vi "CRYAPI SPLITE.vi"(4 "tSpliter_In":T2, 6 "tFrame":T4, 8 "tSpliter":T2, 9 "sData":string, 10 "nData":i32, 11 "sAction":string) -> (0 "nData_Out":i32, 1 "tLR_Out":T1, 3 "tSpliter_Out":T2)   [LabVIEW 2013]
uses:
  <vilib>/Utility/miscctls.llb/LVRectTypeDef.ctl
  CRYMain Sub Window Global.vi
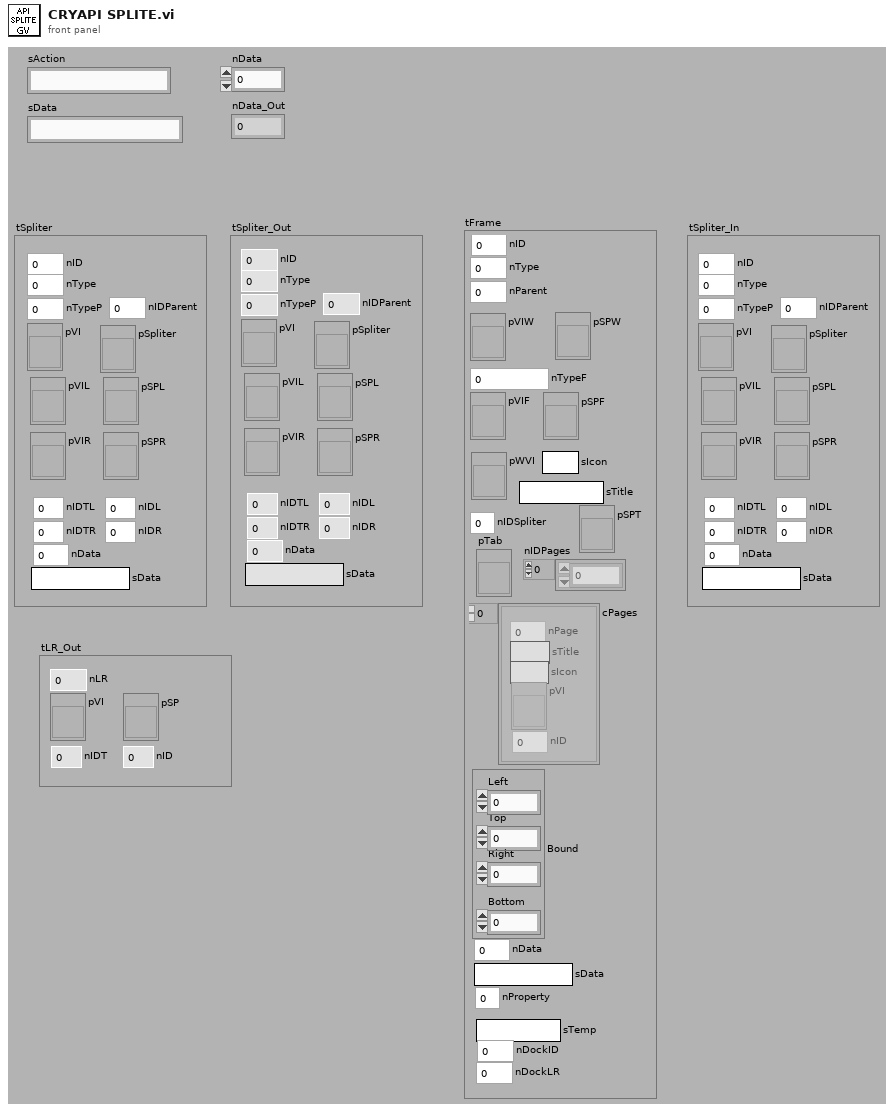
[diagram p1: front panel]
types:
  T1 = cluster{"pSP":refnum<vi>, "pVI":refnum<vi>, "nIDT":i32, "nID":i32, "nLR":i32}
  T2 = cluster{"nType":i32, "nTypeP":i32, "pVI":refnum<vi>, "pSpliter":refnum<vi>, "pSPL":refnum<vi>, "pVIL":refnum<vi>, "pSPR":refnum<vi>, "pVIR":refnum<vi>, "nIDTL":i32, "nIDL":i32, "nIDTR":i32, "nIDR":i32, "nID":i32, "nIDParent":i32, "nData":i32, "sData":string}
  T3 = typedef "LVRectTypeDef.ctl" = cluster{"Left":i16, "Top":i16, "Right":i16, "Bottom":i16}
  T4 = cluster{"nType":i32, "nParent":i32, "pVIW":refnum<vi>, "pSPW":refnum<vi>, "nTypeF":i32, "pVIF":refnum<vi>, "pSPF":refnum<vi>, "nIDSpliter":i32, "nProperty":i32, "Bound":T3, "nID":i32, "nData":i32, "sData":string, "pWVI":refnum<vi>, "sTitle":string, "cPages":cluster{"nPage":i32, "sTitle":string, "sIcon":string, "pVI":refnum<vi>, "nID":i32}[], "pTab":refnum<vi>, "nIDPages":i32[], "pSPT":refnum<vi>, "sTemp":string, "nDockID":i32, "nDockLR":i32, "sIcon":string}
  T5 = enum16{"Sticks Top/Left", "Sticks Bottom/Right", "Proportional"}
  T6 = cluster{"nID":i32, "sTiltle":string, "pVI":refnum<vi>, "pSP":refnum<vi>, "pTab":refnum<vi>, "pSPT":refnum<vi>, "nWinType":i32, "sIcon":string}
  T7 = cluster{"nID":i32[], "Spliter":cluster{"nType":i32, "nTypeP":i32, "pVI":refnum<vi>, "pSpliter":refnum<vi>, "pSPL":refnum<vi>, "pVIL":refnum<vi>, "pSPR":refnum<vi>, "pVIR":refnum<vi>, "nIDTL":i32, "nIDL":i32, "nIDTR":i32, "nIDR":i32, "nID":i32, "nIDParent":i32, "nData":i32, "sData":string}[]}
  T8 = cluster{"nType":i32, "nTypeP":i32, "pVI":refnum<vi>, "pSpliter":refnum<vi>, "pSPL":refnum<vi>, "pVIL":refnum<vi>, "pSPR":refnum<vi>, "pVIR":refnum<vi>, "nIDTL":i32, "nIDL":i32, "nIDTR":i32, "nIDR":i32, "nID":i32, "nIDParent":i32, "nData":i32, "sData":string}[]
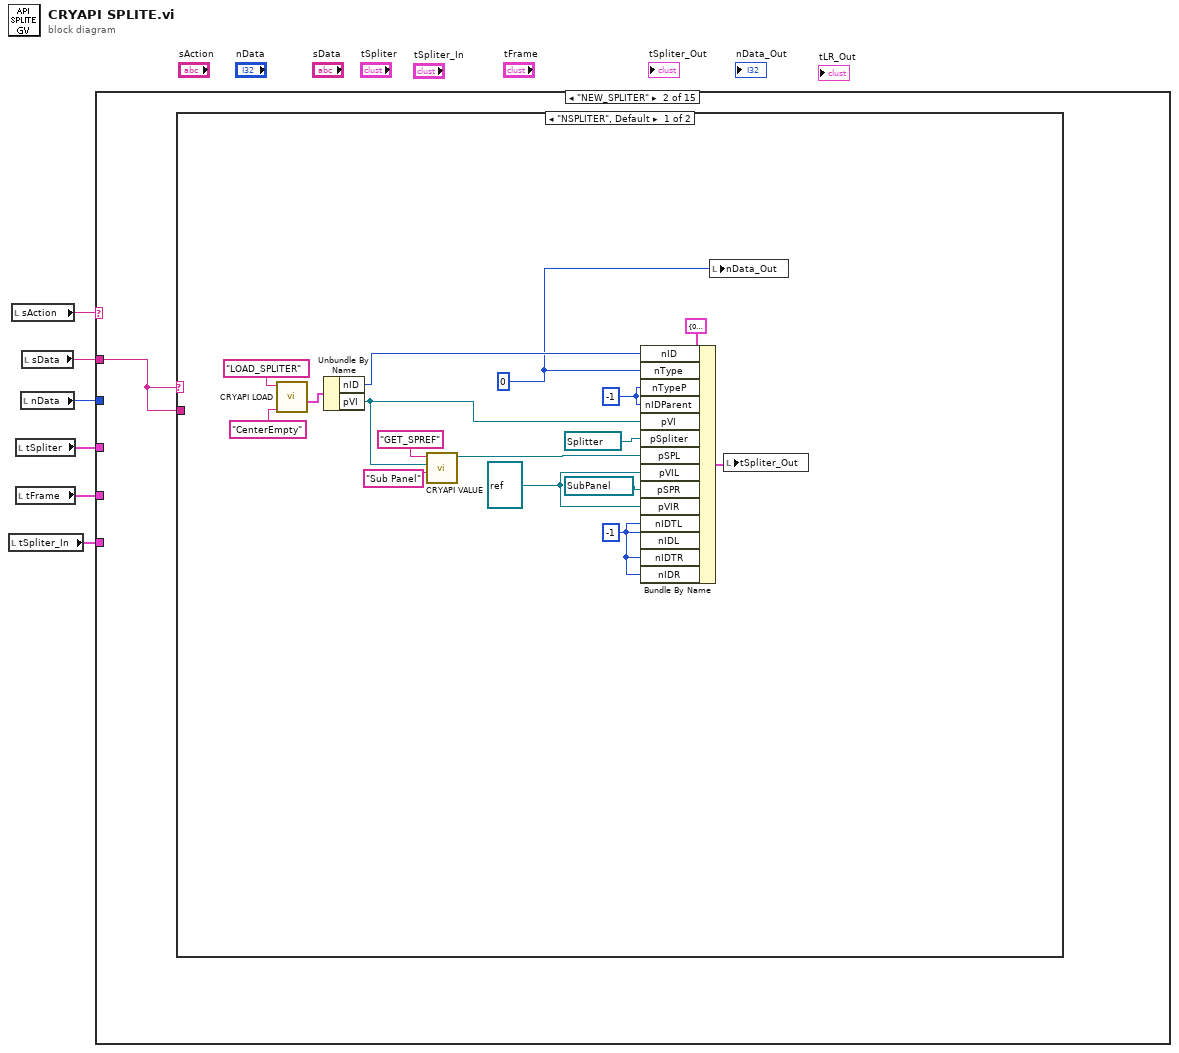
[diagram p0: block diagram]
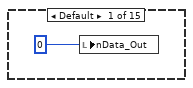
[diagram p2: hidden frame]
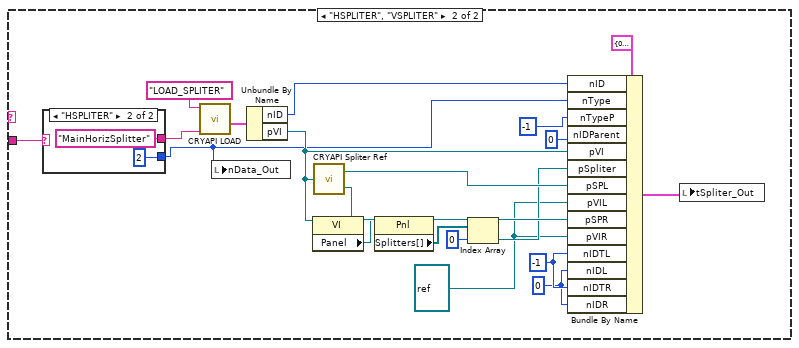
[diagram p3: hidden frame]
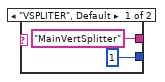
[diagram p4: hidden frame]
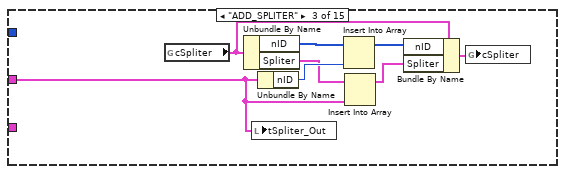
[diagram p5: hidden frame]
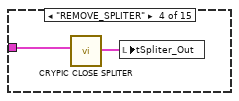
[diagram p6: hidden frame]
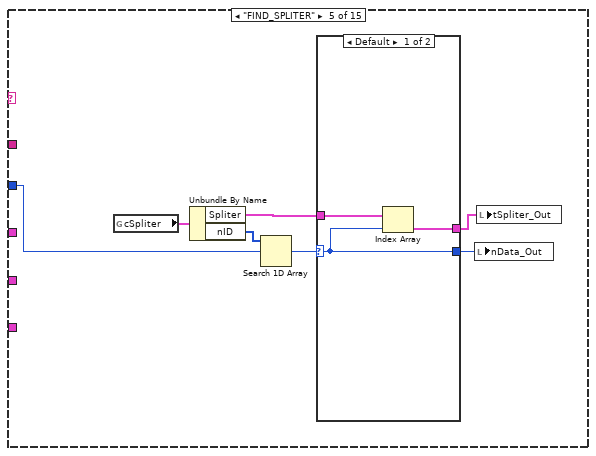
[diagram p7: hidden frame]
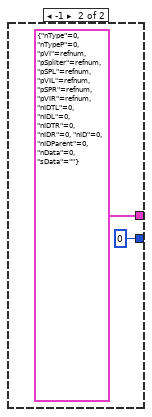
[diagram p8: hidden frame]
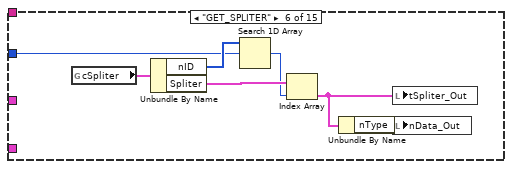
[diagram p9: hidden frame]
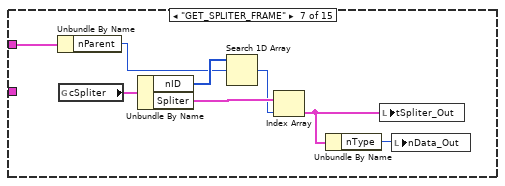
[diagram p10: hidden frame]
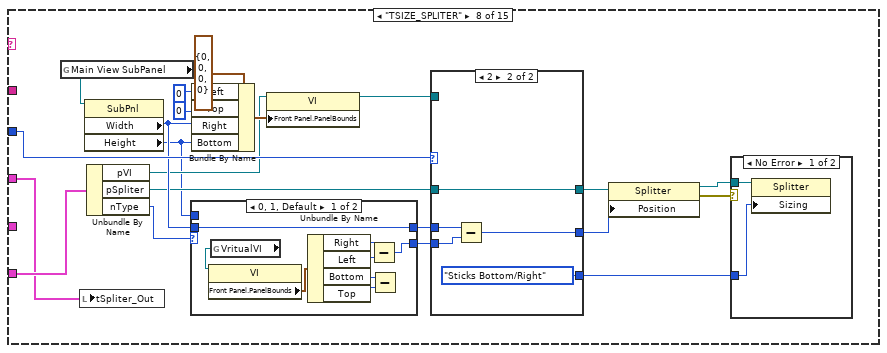
[diagram p11: hidden frame]
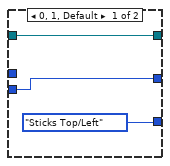
[diagram p13: hidden frame]
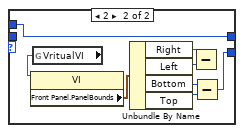
[diagram p14: hidden frame]
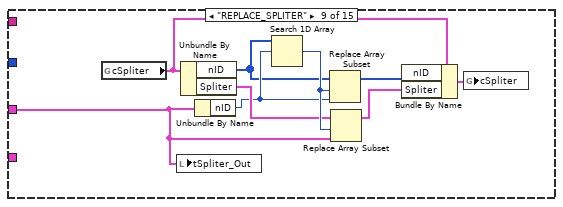
[diagram p15: hidden frame]
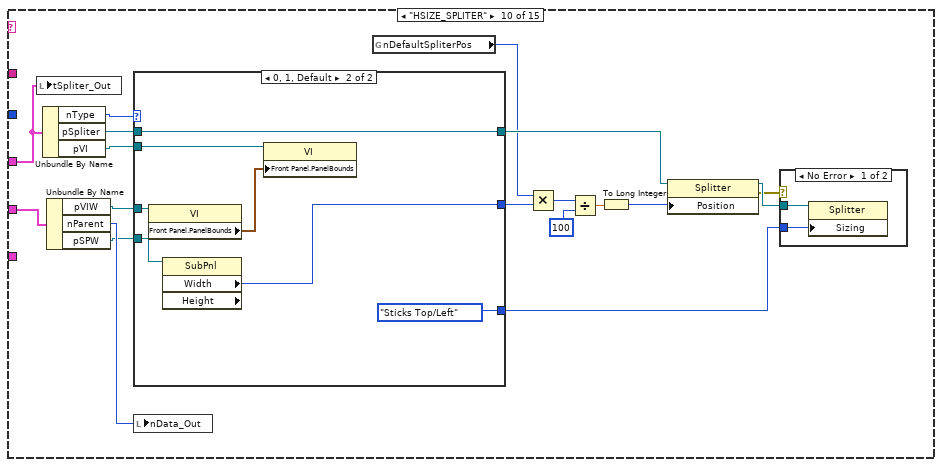
[diagram p16: hidden frame]
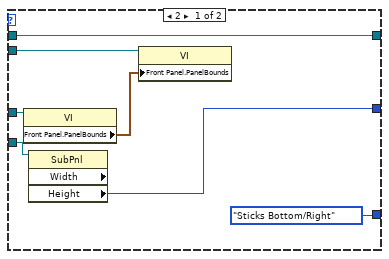
[diagram p18: hidden frame]
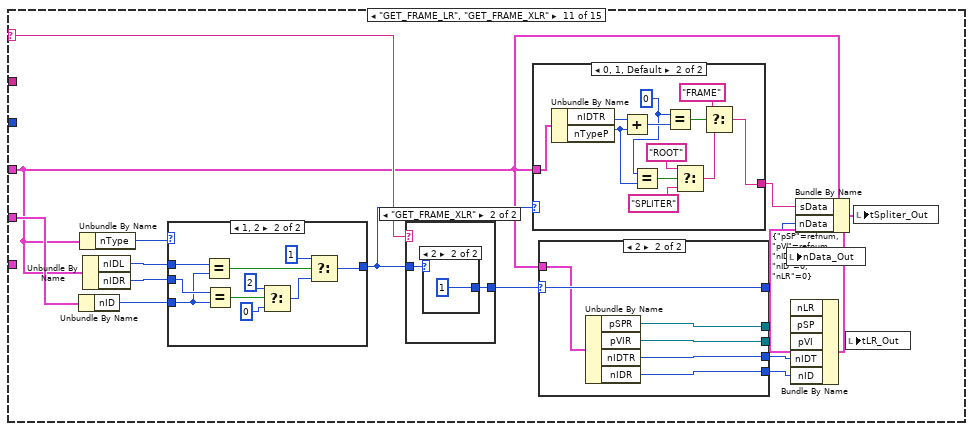
[diagram p19: hidden frame]
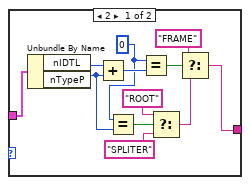
[diagram p20: hidden frame]
diagram:
  n1 = local read "tSpliter_In"() -> (w1:T2)
  n2 = local read "sAction"() -> (w6:string)
  n3 = local read "tSpliter"() -> (w4:T2)
  n4 = local read "tFrame"() -> (w2:T4)
  n5 = local read "nData"() -> (w3:i32)
  n6 = local read "sData"() -> (w5:string)
  n7 = case shown="\"NEW_SPLITER\"" w6 {
    selector: w6 -> [_ _ _ _ _ _ _ _ _ _ w181 w252 w322 w391 _]
    tunnel: w5 -> [_ w8 _ _ _ _ _ _ _ _ _ _ _ w389 w443]
    tunnel: w4 -> [_ _ w49 w58 _ _ _ w86 w133 w156 w176 w248 w319 w390 _]
    tunnel: w3 -> [_ _ _ _ w64 w74 _ w100 _ _ _ _ w316 w388 w448]
    tunnel: w2 -> [_ _ _ _ _ _ w79 _ _ w151 w189 _ _ _ w444]
    tunnel: w1 -> [_ _ _ _ _ _ _ w87 _ _ _ w249 _ _ _]
    frame Default {
      n8 = local write "nData_Out"(0 ("nData_Out")) -> ()
    }
    frame "NEW_SPLITER" {
      n9 = case shown="\"NSPLITER\", Default" w8 {
        tunnel: w8 -> [_ w41]
        frame "NSPLITER", Default {
          w19 = -1
          w20 = refnum<vi> refnum ("pVIL")
          w16 = -1 ("nParent")
          w10 = 0
          n10 = call "CRYAPI LOAD.vi"("sData"="CenterEmpty" ("sAction"), "sAction"="LOAD_SPLITER") -> ("tWindow_Out"=w22:T6)  [unwired: 4 in, 5 out]
          n11 = Unbundle By Name(w22) -> ("nID"=w21:i32, "pVI"=w12:refnum<vi>)
          n12 = call "CRYAPI VALUE.vi"("sControlName"="Sub Panel", "pVIRef"=w12, "sAction"="GET_SPREF") -> ("pSPRef"=w11:refnum<vi>)  [unwired: 2 in, 6 out]
          n13 = Bundle By Name(cluster=T2 {"nType"=0, "nTypeP"=0, "pVI"=refnum, "pSpliter"=refnum, "pSPL"=refnum, "pVIL"=refnum, "pSPR"=refnum, "pVIR"=refnum, "nIDTL"=0, "nIDL"=0, "nIDTR"=0, "nIDR"=0, "nID"=0, "nIDParent"=0, "nData"=0, "sData"=""} ("tSpliter_Out"), "nID"=w21, "nType"=w10, "nTypeP"=w16, "nIDParent"=w16, "pVI"=w12, "pSpliter"=refnum<vi> refnum, "pSPL"=w11, "pVIL"=w20, "pSPR"=refnum<vi> refnum, "pVIR"=w20, "nIDTL"=w19, "nIDL"=w19, "nIDTR"=w19, "nIDR"=w19) -> (w24:T2)
          n14 = local write "nData_Out"(w10) -> ()
          n15 = local write "tSpliter_Out"(w24) -> ()
        }
        frame "HSPLITER", "VSPLITER" {
          w28 = 0
          w32 = -1
          w33 = refnum<vi> refnum ("pVIL")
          n16 = case shown="\"HSPLITER\"" w41 {
            tunnel: ["MainVertSplitter" ("sAction") "MainHorizSplitter" ("sAction")] -> w42
            tunnel: [1 2] -> w29
            frame "VSPLITER", Default {
            }
            frame "HSPLITER" {
            }
          }
          n17 = call "CRYAPI LOAD.vi"("sData"=w42, "sAction"="LOAD_SPLITER") -> ("tWindow_Out"=w43:T6)  [unwired: 4 in, 5 out]
          n18 = local write "nData_Out"(w29) -> ()
          n19 = Unbundle By Name(w43) -> ("nID"=w34:i32, "pVI"=w31:refnum<vi>)
          n20 = property class="VI"(reference=w31) -> ("Panel"=w36:refnum<vi>)  [unwired: 1 in, 2 out]
          n21 = call "CRYAPI Spliter Ref.vi"("VI Refnum"=w31) -> ("Left/Upper"=w40:refnum<vi>, "Right/Lower"=w39:refnum<vi>)
          n22 = property class="Pnl"(reference=w36) -> ("Splitters[]"=w37:refnum<vi>[])  [unwired: 1 in, 2 out]
          n23 = Index Array(array=w37, index=0) -> (element=w35:refnum<vi>)
          n24 = Bundle By Name(cluster=T2 {"nType"=0, "nTypeP"=0, "pVI"=refnum, "pSpliter"=refnum, "pSPL"=refnum, "pVIL"=refnum, "pSPR"=refnum, "pVIR"=refnum, "nIDTL"=0, "nIDL"=0, "nIDTR"=0, "nIDR"=0, "nID"=0, "nIDParent"=0, "nData"=0, "sData"=""} ("tSpliter_Out"), "nID"=w34, "nType"=w29, "nTypeP"=-1 ("nParent"), "nIDParent"=0 ("nParent"), "pVI"=w31, "pSpliter"=w35, "pSPL"=w40, "pVIL"=w33, "pSPR"=w39, "pVIR"=w33, "nIDTL"=w32, "nIDL"=w28, "nIDTR"=w32, "nIDR"=w28) -> (w25:T2)
          n25 = local write "tSpliter_Out"(w25) -> ()
        }
      }
    }
    frame "ADD_SPLITER" {
      n26 = global read "CRYMain Sub Window Global.vi" "cSpliter"() -> (w53:T7)
      n27 = Unbundle By Name(w53) -> ("nID"=w50:i32[], "Spliter"=w51:T8)
      n28 = local write "tSpliter_Out"(w49) -> ()
      n29 = Unbundle By Name(w49) -> ("nID"=w52:i32)
      n30 = Insert Into Array(array=w50, new element=w52) -> (w54:i32[])  [unwired: 1 in]
      n31 = Insert Into Array(array=w51, new element=w49) -> (w55:T8)  [unwired: 1 in]
      n32 = Bundle By Name(cluster=w53, "nID"=w54, "Spliter"=w55) -> (w56:T7)
      n33 = global write "CRYMain Sub Window Global.vi" "cSpliter"(w56) -> ()
    }
    frame "REMOVE_SPLITER" {
      n34 = call "CRYPIC CLOSE SPLITER.vi"("tSpliter"=w58) -> ("tSpliter_Out"=w57:T2)  [unwired: 10 in]
      n35 = local write "tSpliter_Out"(w57) -> ()
    }
    frame "FIND_SPLITER" {
      n36 = global read "CRYMain Sub Window Global.vi" "cSpliter"() -> (w62:T7)
      n37 = Unbundle By Name(w62) -> ("Spliter"=w61:T8, "nID"=w65:i32[])
      n38 = Search 1D Array(1D array=w65, element=w64) -> (index of element=w63:i32)  [unwired: 1 out]
      n39 = case shown="Default" w63 {
        selector: w63 -> [w66 _]
        tunnel: w61 -> [w68 _]
        tunnel: [w67 T2 {"nType"=0, "nTypeP"=0, "pVI"=refnum, "pSpliter"=refnum, "pSPL"=refnum, "pVIL"=refnum, "pSPR"=refnum, "pVIR"=refnum, "nIDTL"=0, "nIDL"=0, "nIDTR"=0, "nIDR"=0, "nID"=0, "nIDParent"=0, "nData"=0, "sData"=""} ("tSpliter")] -> w59
        tunnel: [w66 0 ("index of element")] -> w60
        frame Default {
          n40 = Index Array(array=w68, index=w66) -> (element=w67:T2)
        }
        frame -1 {
        }
      }
      n41 = local write "nData_Out"(w60) -> ()
      n42 = local write "tSpliter_Out"(w59) -> ()
    }
    frame "GET_SPLITER" {
      n43 = global read "CRYMain Sub Window Global.vi" "cSpliter"() -> (w77:T7)
      n44 = Unbundle By Name(w77) -> ("nID"=w75:i32[], "Spliter"=w76:T8)
      n45 = Search 1D Array(1D array=w75, element=w74) -> (index of element=w73:i32)  [unwired: 1 out]
      n46 = Index Array(array=w76, index=w73) -> (element=w72:T2)
      n47 = Unbundle By Name(w72) -> ("nType"=w71:i32)
      n48 = local write "tSpliter_Out"(w72) -> ()
      n49 = local write "nData_Out"(w71) -> ()
    }
    frame "GET_SPLITER_FRAME" {
      n50 = Unbundle By Name(w79) -> ("nParent"=w78:i32)
      n51 = global read "CRYMain Sub Window Global.vi" "cSpliter"() -> (w85:T7)
      n52 = Unbundle By Name(w85) -> ("nID"=w83:i32[], "Spliter"=w84:T8)
      n53 = Search 1D Array(1D array=w83, element=w78) -> (index of element=w82:i32)  [unwired: 1 out]
      n54 = Index Array(array=w84, index=w82) -> (element=w81:T2)
      n55 = Unbundle By Name(w81) -> ("nType"=w80:i32)
      n56 = local write "tSpliter_Out"(w81) -> ()
      n57 = local write "nData_Out"(w80) -> ()
    }
    frame "TSIZE_SPLITER" {
      n58 = global read "CRYMain Sub Window Global.vi" "Main View SubPanel"() -> (w106:refnum<vi>)
      n59 = local write "tSpliter_Out"(w86) -> ()
      n60 = property class="SubPnl"(reference=w106) -> ("Width"=w98:u32, "Height"=w93:u32)  [unwired: 1 in, 2 out]
      n61 = Unbundle By Name(w87) -> ("pVI"=w95:refnum<vi>, "pSpliter"=w94:refnum<vi>, "nType"=w101:i32)
      n62 = case shown="0, 1, Default" w101 {
        tunnel: [w118 w126] -> w99
        tunnel: w93 -> [_ w125]
        tunnel: w98 -> [w117 _]
        tunnel: [w117 w125] -> w97
        frame 0, 1, Default {
          n63 = global read "CRYMain Sub Window Global.vi" "VritualVI"() -> (w124:refnum<vi>)
          n64 = property class="VI"(reference=w124) -> ("Front Panel.PanelBounds"=w123:T3)  [unwired: 1 in, 2 out]
          n65 = Unbundle By Name(w123) -> ("Right"=w122:i16, "Left"=w121:i16, "Bottom"=w120:i16, "Top"=w119:i16)
          n66 = Subtract(x=w122, y=w121) -> (x-y=w118:i16)
          n67 = Subtract(x=w120, y=w119) -> ()  [unwired: 1 out]
        }
        frame 2 {
          n68 = global read "CRYMain Sub Window Global.vi" "VritualVI"() -> (w132:refnum<vi>)
          n69 = property class="VI"(reference=w132) -> ("Front Panel.PanelBounds"=w131:T3)  [unwired: 1 in, 2 out]
          n70 = Unbundle By Name(w131) -> ("Right"=w130:i16, "Left"=w129:i16, "Bottom"=w128:i16, "Top"=w127:i16)
          n71 = Subtract(x=w130, y=w129) -> ()  [unwired: 1 out]
          n72 = Subtract(x=w128, y=w127) -> (x-y=w126:i16)
        }
      }
      n73 = Bundle By Name(cluster=T3 {"Left"=0, "Top"=0, "Right"=0, "Bottom"=0} ("Bound_Out"), "Left"=i16 0, "Top"=i16 0, "Right"=w98, "Bottom"=w93) -> (w105:T3)
      n74 = property class="VI"(reference=w95, "Front Panel.PanelBounds"=w105) -> (reference out=w96:refnum<vi>)  [unwired: 1 in, 1 out]
      n75 = case shown="2" w100 {
        tunnel: w99 -> [w111 w115]
        tunnel: [w111 w114] -> w91
        tunnel: w97 -> [_ w116]
        tunnel: w96 -> [_ _]
        tunnel: w94 -> [w110 w113]
        tunnel: [w110 w113] -> w92
        tunnel: [T5."Sticks Top/Left" ("Sizing") T5."Sticks Bottom/Right" ("Sizing")] -> w88
        frame 0, 1, Default {
        }
        frame 2 {
          n76 = Subtract(x=w116, y=w115) -> (x-y=w114:u32)
        }
      }
      n77 = property class="Splitter"(reference=w92, "Position"=w91) -> (reference out=w89:refnum<vi>, error out=w90:errorcluster)  [unwired: 1 in]
      n78 = case shown="No Error" w90 {
        tunnel: w88 -> [w108 _]
        tunnel: w89 -> [w107 _]
        frame No Error {
          n79 = property class="Splitter"(reference=w107, "Sizing"=w108) -> ()  [unwired: 1 in, 2 out]
        }
        frame Error {
        }
      }
    }
    frame "REPLACE_SPLITER" {
      n80 = global read "CRYMain Sub Window Global.vi" "cSpliter"() -> (w136:T7)
      n81 = local write "tSpliter_Out"(w133) -> ()
      n82 = Unbundle By Name(w136) -> ("nID"=w137:i32[], "Spliter"=w140:T8)
      n83 = Unbundle By Name(w133) -> ("nID"=w138:i32)
      n84 = Search 1D Array(1D array=w137, element=w138) -> (index of element=w141:i32)  [unwired: 1 out]
      n85 = Replace Array Subset(array=w137, new element=w138, index=w141) -> (w135:i32[])
      n86 = Replace Array Subset(array=w140, new element=w133, index=w141) -> (w139:T8)
      n87 = Bundle By Name(cluster=w136, "nID"=w135, "Spliter"=w139) -> (w134:T7)
      n88 = global write "CRYMain Sub Window Global.vi" "cSpliter"(w134) -> ()
    }
    frame "HSIZE_SPLITER" {
      n89 = local write "tSpliter_Out"(w156) -> ()
      n90 = Unbundle By Name(w156) -> ("nType"=w152:i32, "pSpliter"=w154:refnum<vi>, "pVI"=w155:refnum<vi>)
      n91 = Unbundle By Name(w151) -> ("pVIW"=w159:refnum<vi>, "nParent"=w150:i32, "pSPW"=w149:refnum<vi>)
      n92 = case shown="0, 1, Default" w152 {
        tunnel: w159 -> [w168 w175]
        tunnel: [w163 w170] -> w146
        tunnel: w155 -> [w167 w174]
        tunnel: w154 -> [w165 w172]
        tunnel: [w165 w172] -> w153
        tunnel: w149 -> [w164 w171]
        tunnel: [T5."Sticks Bottom/Right" ("Sizing") T5."Sticks Top/Left" ("Sizing")] -> w148
        frame 2 {
          n93 = property class="VI"(reference=w168) -> ("Front Panel.PanelBounds"=w166:T3)  [unwired: 1 in, 2 out]
          n94 = property class="SubPnl" props=["Width", "Height"](reference=w164) -> ("Height"=w163:u32)  [unwired: 1 in, 3 out]
          n95 = property class="VI"(reference=w167, "Front Panel.PanelBounds"=w166) -> ()  [unwired: 1 in, 2 out]
        }
        frame 0, 1, Default {
          n96 = property class="VI"(reference=w175) -> ("Front Panel.PanelBounds"=w173:T3)  [unwired: 1 in, 2 out]
          n97 = property class="SubPnl" props=["Width", "Height"](reference=w171) -> ("Width"=w170:u32)  [unwired: 1 in, 3 out]
          n98 = property class="VI"(reference=w174, "Front Panel.PanelBounds"=w173) -> ()  [unwired: 1 in, 2 out]
        }
      }
      n99 = local write "nData_Out"(w150) -> ()
      n100 = global read "CRYMain Sub Window Global.vi" "nDefaultSpliterPos"() -> (w147:i32)
      n101 = Multiply(x=w147, y=w146) -> (x*y=w145:u32)
      n102 = Divide(x=w145, y=u32 100) -> (x/y=w143:dbl)
      n103 = To Long Integer(number=w143) -> (32bit integer=w142:i32)
      n104 = property class="Splitter"(reference=w153, "Position"=w142) -> (reference out=w158:refnum<vi>, error out=w157:errorcluster)  [unwired: 1 in]
      n105 = case shown="No Error" w157 {
        tunnel: w158 -> [w161 _]
        tunnel: w148 -> [w160 _]
        frame No Error {
          n106 = property class="Splitter"(reference=w161, "Sizing"=w160) -> ()  [unwired: 1 in, 2 out]
        }
        frame Error {
        }
      }
    }
    frame "GET_FRAME_LR", "GET_FRAME_XLR" {
      n107 = Unbundle By Name(w189) -> ("nID"=w191:i32)
      n108 = Unbundle By Name(w176) -> ("nType"=w190:i32)
      n109 = Unbundle By Name(w176) -> ("nIDL"=w192:i32, "nIDR"=w193:i32)
      n110 = case shown="1, 2" w190 {
        tunnel: w191 -> [_ w243]
        tunnel: w192 -> [_ w245]
        tunnel: w193 -> [_ w244]
        tunnel: [0 w236] -> w178
        frame 0, Default {
        }
        frame 1, 2 {
          n111 = Equal?(x=w245, y=w243) -> (x = y?=w242:bool)
          n112 = Equal?(x=w244, y=w243) -> (x = y?=w239:bool)
          n113 = Select(t=2, s=w239, f=0) -> (s? t:f=w240:i32)
          n114 = Select(t=1, s=w242, f=w240) -> (s? t:f=w236:i32)
        }
      }
      n115 = case shown="\"GET_FRAME_XLR\"" w181 {
        tunnel: w178 -> [w218 w220]
        tunnel: [w218 w219] -> w179
        frame "GET_FRAME_LR", Default {
        }
        frame "GET_FRAME_XLR" {
          n116 = case shown="2" w220 {
            tunnel: [2 1] -> w219
            frame 0, 1, Default {
            }
            frame 2 {
            }
          }
        }
      }
      n117 = case shown="0, 1, Default" w178 {
        tunnel: w176 -> [w203 w215]
        tunnel: [w202 w214] -> w177
        frame 2 {
          w200 = 0 ("y")
          n118 = Unbundle By Name(w203) -> ("nIDTL"=w197:i32, "nTypeP"=w196:i32)
          n119 = Add(x=w197, y=w196) -> (x+y=w201:i32)
          n120 = Equal?(x=w200, y=w196) -> (x = y?=w199:bool)
          n121 = Equal?(x=w200, y=w201) -> (x = y?=w205:bool)
          n122 = Select(t="ROOT", s=w199, f="SPLITER") -> (s? t:f=w198:string)
          n123 = Select(t="FRAME", s=w205, f=w198) -> (s? t:f=w202:string)
        }
        frame 0, 1, Default {
          w212 = 0 ("y")
          n124 = Unbundle By Name(w215) -> ("nIDTR"=w209:i32, "nTypeP"=w208:i32)
          n125 = Add(x=w209, y=w208) -> (x+y=w213:i32)
          n126 = Equal?(x=w212, y=w208) -> (x = y?=w211:bool)
          n127 = Equal?(x=w212, y=w213) -> (x = y?=w217:bool)
          n128 = Select(t="ROOT", s=w211, f="SPLITER") -> (s? t:f=w210:string)
          n129 = Select(t="FRAME", s=w217, f=w210) -> (s? t:f=w214:string)
        }
      }
      n130 = case shown="2" w179 {
        selector: w179 -> [w224 w230]
        tunnel: w176 -> [w223 w229]
        tunnel: [w228 w234] -> w186
        tunnel: [w227 w233] -> w185
        tunnel: [w226 w232] -> w184
        tunnel: [w225 w231] -> w183
        tunnel: [w224 w230] -> w180
        frame 0, 1, Default {
          n131 = Unbundle By Name(w223) -> ("pSPL"=w228:refnum<vi>, "pVIL"=w227:refnum<vi>, "nIDTL"=w226:i32, "nIDL"=w225:i32)
        }
        frame 2 {
          n132 = Unbundle By Name(w229) -> ("pSPR"=w234:refnum<vi>, "pVIR"=w233:refnum<vi>, "nIDTR"=w232:i32, "nIDR"=w231:i32)
        }
      }
      n133 = local write "nData_Out"(w180) -> ()
      n134 = Bundle By Name(cluster=T1 {"pSP"=refnum, "pVI"=refnum, "nIDT"=0, "nID"=0, "nLR"=0} ("tLR_Out"), "nLR"=w180, "pSP"=w186, "pVI"=w185, "nIDT"=w184, "nID"=w183) -> (w182:T1)
      n135 = Bundle By Name(cluster=w176, "sData"=w177, "nData"=w180) -> (w188:T2)
      n136 = local write "tLR_Out"(w182) -> ()
      n137 = local write "tSpliter_Out"(w188) -> ()
    }
    frame "GET_SPLITER_LR", "GET_SPLITER_XLR" {
      n138 = Unbundle By Name(w249) -> ("nID"=w261:i32)
      n139 = Unbundle By Name(w248) -> ("nType"=w260:i32)
      n140 = Unbundle By Name(w248) -> ("nIDL"=w262:i32, "nIDR"=w263:i32)
      n141 = case shown="1, 2" w260 {
        tunnel: w261 -> [_ w313]
        tunnel: w262 -> [_ w315]
        tunnel: w263 -> [_ w314]
        tunnel: [0 w306] -> w247
        frame 0, Default {
        }
        frame 1, 2 {
          n142 = Equal?(x=w315, y=w313) -> (x = y?=w312:bool)
          n143 = Equal?(x=w314, y=w313) -> (x = y?=w309:bool)
          n144 = Select(t=2, s=w309, f=0) -> (s? t:f=w310:i32)
          n145 = Select(t=1, s=w312, f=w310) -> (s? t:f=w306:i32)
        }
      }
      n146 = case shown="\"GET_SPLITER_XLR\"" w252 {
        tunnel: w247 -> [w288 w290]
        tunnel: [w288 w289] -> w250
        frame "GET_SPLITER_LR", Default {
        }
        frame "GET_SPLITER_XLR" {
          n147 = case shown="2" w290 {
            tunnel: [2 1] -> w289
            frame 0, 1, Default {
            }
            frame 2 {
            }
          }
        }
      }
      n148 = case shown="0, 1, Default" w247 {
        tunnel: w248 -> [w273 w285]
        tunnel: [w272 w284] -> w246
        frame 2 {
          w270 = 0 ("y")
          n149 = Unbundle By Name(w273) -> ("nIDTL"=w267:i32, "nTypeP"=w266:i32)
          n150 = Add(x=w267, y=w266) -> (x+y=w271:i32)
          n151 = Equal?(x=w270, y=w266) -> (x = y?=w269:bool)
          n152 = Equal?(x=w270, y=w271) -> (x = y?=w275:bool)
          n153 = Select(t="ROOT", s=w269, f="SPLITER") -> (s? t:f=w268:string)
          n154 = Select(t="FRAME", s=w275, f=w268) -> (s? t:f=w272:string)
        }
        frame 0, 1, Default {
          w282 = 0 ("y")
          n155 = Unbundle By Name(w285) -> ("nIDTR"=w279:i32, "nTypeP"=w278:i32)
          n156 = Add(x=w279, y=w278) -> (x+y=w283:i32)
          n157 = Equal?(x=w282, y=w278) -> (x = y?=w281:bool)
          n158 = Equal?(x=w282, y=w283) -> (x = y?=w287:bool)
          n159 = Select(t="ROOT", s=w281, f="SPLITER") -> (s? t:f=w280:string)
          n160 = Select(t="FRAME", s=w287, f=w280) -> (s? t:f=w284:string)
        }
      }
      n161 = case shown="2" w250 {
        selector: w250 -> [w294 w300]
        tunnel: w248 -> [w293 w299]
        tunnel: [w298 w304] -> w257
        tunnel: [w297 w303] -> w256
        tunnel: [w296 w302] -> w255
        tunnel: [w295 w301] -> w254
        tunnel: [w294 w300] -> w251
        frame 0, 1, Default {
          n162 = Unbundle By Name(w293) -> ("pSPL"=w298:refnum<vi>, "pVIL"=w297:refnum<vi>, "nIDTL"=w296:i32, "nIDL"=w295:i32)
        }
        frame 2 {
          n163 = Unbundle By Name(w299) -> ("pSPR"=w304:refnum<vi>, "pVIR"=w303:refnum<vi>, "nIDTR"=w302:i32, "nIDR"=w301:i32)
        }
      }
      n164 = local write "nData_Out"(w251) -> ()
      n165 = Bundle By Name(cluster=T1 {"pSP"=refnum, "pVI"=refnum, "nIDT"=0, "nID"=0, "nLR"=0} ("tLR_Out"), "nLR"=w251, "pSP"=w257, "pVI"=w256, "nIDT"=w255, "nID"=w254) -> (w253:T1)
      n166 = Bundle By Name(cluster=w248, "sData"=w246, "nData"=w251) -> (w259:T2)
      n167 = local write "tLR_Out"(w253) -> ()
      n168 = local write "tSpliter_Out"(w259) -> ()
    }
    frame "GET_ID_LR", "GET_ID_XLR" {
      n169 = Unbundle By Name(w319) -> ("nType"=w330:i32)
      n170 = Unbundle By Name(w319) -> ("nIDL"=w331:i32, "nIDR"=w332:i32)
      n171 = case shown="0, Default" w330 {
        tunnel: w316 -> [_ w383]
        tunnel: w331 -> [_ w385]
        tunnel: w332 -> [_ w384]
        tunnel: [0 w376] -> w318
        frame 0, Default {
        }
        frame 1, 2 {
          n172 = Equal?(x=w385, y=w383) -> (x = y?=w382:bool)
          n173 = Equal?(x=w384, y=w383) -> (x = y?=w379:bool)
          n174 = Select(t=2, s=w379, f=0) -> (s? t:f=w380:i32)
          n175 = Select(t=1, s=w382, f=w380) -> (s? t:f=w376:i32)
        }
      }
      n176 = case shown="\"GET_ID_XLR\"" w322 {
        tunnel: w318 -> [w357 w359]
        tunnel: [w357 w358] -> w320
        frame "GET_ID_LR", Default {
        }
        frame "GET_ID_XLR" {
          n177 = case shown="0, Default" w359 {
            selector: w359 -> [w360 _ _]
            tunnel: [w360 2 1] -> w358
            frame 0, Default {
            }
            frame 1 {
            }
            frame 2 {
            }
          }
        }
      }
      n178 = case shown="0, 1, Default" w318 {
        tunnel: w319 -> [w342 w354]
        tunnel: [w341 w353] -> w317
        frame 2 {
          w339 = 0 ("y")
          n179 = Unbundle By Name(w342) -> ("nIDTL"=w336:i32, "nTypeP"=w335:i32)
          n180 = Add(x=w336, y=w335) -> (x+y=w340:i32)
          n181 = Equal?(x=w339, y=w335) -> (x = y?=w338:bool)
          n182 = Equal?(x=w339, y=w340) -> (x = y?=w344:bool)
          n183 = Select(t="ROOT", s=w338, f="SPLITER") -> (s? t:f=w337:string)
          n184 = Select(t="FRAME", s=w344, f=w337) -> (s? t:f=w341:string)
        }
        frame 0, 1, Default {
          w351 = 0 ("y")
          n185 = Unbundle By Name(w354) -> ("nIDTR"=w348:i32, "nTypeP"=w347:i32)
          n186 = Add(x=w348, y=w347) -> (x+y=w352:i32)
          n187 = Equal?(x=w351, y=w347) -> (x = y?=w350:bool)
          n188 = Equal?(x=w351, y=w352) -> (x = y?=w356:bool)
          n189 = Select(t="ROOT", s=w350, f="SPLITER") -> (s? t:f=w349:string)
          n190 = Select(t="FRAME", s=w356, f=w349) -> (s? t:f=w353:string)
        }
      }
      n191 = case shown="0, 1, Default" w320 {
        selector: w320 -> [w364 w370]
        tunnel: w319 -> [w363 w369]
        tunnel: [w368 w374] -> w327
        tunnel: [w367 w373] -> w326
        tunnel: [w366 w372] -> w325
        tunnel: [w365 w371] -> w324
        tunnel: [w364 w370] -> w321
        frame 0, 1, Default {
          n192 = Unbundle By Name(w363) -> ("pSPL"=w368:refnum<vi>, "pVIL"=w367:refnum<vi>, "nIDTL"=w366:i32, "nIDL"=w365:i32)
        }
        frame 2 {
          n193 = Unbundle By Name(w369) -> ("pSPR"=w374:refnum<vi>, "pVIR"=w373:refnum<vi>, "nIDTR"=w372:i32, "nIDR"=w371:i32)
        }
      }
      n194 = local write "nData_Out"(w321) -> ()
      n195 = Bundle By Name(cluster=T1 {"pSP"=refnum, "pVI"=refnum, "nIDT"=0, "nID"=0, "nLR"=0} ("tLR_Out"), "nLR"=w321, "pSP"=w327, "pVI"=w326, "nIDT"=w325, "nID"=w324) -> (w323:T1)
      n196 = Bundle By Name(cluster=w319, "sData"=w317, "nData"=w321) -> (w329:T2)
      n197 = local write "tLR_Out"(w323) -> ()
      n198 = local write "tSpliter_Out"(w329) -> ()
    }
    frame "GET_LR_INDEX", "GET_XLR_INDEX" {
      n199 = Equal?(x=w388, y=-1) -> (x = y?=w386:bool)
      n200 = case shown="False" w386 {
        tunnel: w391 -> [w405 _]
        tunnel: w390 -> [w403 w439]
        tunnel: w388 -> [w398 _]
        tunnel: w389 -> [w397 _]
        frame False {
          n201 = Unbundle By Name(w403) -> ("nType"=w402:i32)
          n202 = case shown="\"VSPLITER\"" w397 {
            tunnel: [2 1] -> w396
            frame "HSPLITER", Default {
            }
            frame "VSPLITER" {
            }
          }
          n203 = case shown="\"GET_LR_INDEX\", Default" w405 {
            tunnel: [w419 w421] -> w395
            tunnel: w398 -> [w419 w420]
            frame "GET_LR_INDEX", Default {
            }
            frame "GET_XLR_INDEX" {
              n204 = case shown="2" w420 {
                tunnel: [0 2 1] -> w421
                frame 0, Default {
                }
                frame 1 {
                }
                frame 2 {
                }
              }
            }
          }
          n205 = Equal?(x=w396, y=w402) -> (x = y?=w401:bool)
          n206 = Select(t="==VH", s=w401, f="!=VH") -> (s? t:f=w394:string)
          n207 = case shown="0, 1, Default" w395 {
            selector: w395 -> [w430 w436]
            tunnel: w403 -> [w429 w435]
            tunnel: [w430 w436] -> w406
            tunnel: [w428 w434] -> w411
            tunnel: [w427 w433] -> w410
            tunnel: [w426 w432] -> w409
            tunnel: [w425 w431] -> w408
            frame 2 {
              n208 = Unbundle By Name(w429) -> ("pSPR"=w428:refnum<vi>, "pVIR"=w427:refnum<vi>, "nIDTR"=w426:i32, "nIDR"=w425:i32)
            }
            frame 0, 1, Default {
              n209 = Unbundle By Name(w435) -> ("pSPL"=w434:refnum<vi>, "pVIL"=w433:refnum<vi>, "nIDTL"=w432:i32, "nIDL"=w431:i32)
            }
          }
          n210 = case shown="\"=VH\", Default" w394 {
            selector: w394 -> [w414 w416]
            tunnel: w395 -> [w413 _]
            tunnel: [w414 w416] -> w393
            tunnel: [w413 0] -> w392
            frame "==VH" {
            }
            frame "=VH", Default {
            }
          }
          n211 = Bundle By Name(cluster=w403, "nData"=w392, "sData"=w393) -> (w404:T2)
          n212 = local write "nData_Out"(w406) -> ()
          n213 = Bundle By Name(cluster=T1 {"pSP"=refnum, "pVI"=refnum, "nIDT"=0, "nID"=0, "nLR"=0} ("tLR_Out"), "nLR"=w406, "pSP"=w411, "pVI"=w410, "nIDT"=w409, "nID"=w408) -> (w407:T1)
          n214 = local write "tSpliter_Out"(w404) -> ()
          n215 = local write "tLR_Out"(w407) -> ()
        }
        frame True {
          n216 = Bundle By Name(cluster=w439, "nData"=0, "sData"="!=VH") -> (w440:T2)
          n217 = local write "tSpliter_Out"(w440) -> ()
        }
      }
    }
    frame "MSG_SEND" {
      n218 = case shown="\"CHANGE_PARENT\", \"CLOSE_PAGE\", \"FLOAT_PAGE\"" w443 {
        selector: w443 -> [_ _ _ w468]
        tunnel: w448 -> [_ w459 _ w474]
        tunnel: [refnum<vi> refnum ("MsgProVI") w458 w465 w475] -> w447
        tunnel: w443 -> [w456 w457 _ _]
        tunnel: [w456 w457 "CLOSE_VI" ("Control Name") w468] -> w445
        tunnel: w444 -> [_ _ w464 w470]
        frame "False", Default {
        }
        frame "CLOSE_FRAME", "REMOVE_FRAME_ID", "ToVIEWActive" {
          n219 = global read "CRYMain Sub Window Global.vi" "MsgProVI"() -> (w461:refnum<vi>)
          n220 = invoke class="VI" method="Ctrl Val.Set"(reference=w461, "Control Name"="nData", "Value"=w459) -> (reference out=w458:refnum<vi>)  [unwired: 2 in, 4 out]
        }
        frame "CLOSE_VIF" {
          n221 = global read "CRYMain Sub Window Global.vi" "MsgProVI"() -> (w467:refnum<vi>)
          n222 = Unbundle By Name(w464) -> ("pVIF"=w463:refnum<vi>)
          n223 = invoke class="VI" method="Ctrl Val.Set"(reference=w467, "Control Name"="pVI", "Value"=w463) -> (reference out=w465:refnum<vi>)  [unwired: 2 in, 4 out]
        }
        frame "CHANGE_PARENT", "CLOSE_PAGE", "FLOAT_PAGE" {
          n224 = global read "CRYMain Sub Window Global.vi" "MsgProVI"() -> (w471:refnum<vi>)
          n225 = Unbundle By Name(w470) -> ("nID"=w469:i32)
          n226 = invoke class="VI" method="Ctrl Val.Set"(reference=w471, "Control Name"="nDData", "Value"=w469) -> ()  [unwired: 2 in, 5 out]
          n227 = invoke class="VI" method="Ctrl Val.Set"(reference=w471, "Control Name"="nSData", "Value"=w474) -> (reference out=w475:refnum<vi>)  [unwired: 2 in, 4 out]
        }
      }
      n228 = invoke class="VI" method="Ctrl Val.Set"(reference=w447, "Control Name"="sMsgCommand", "Value"=w445) -> (reference out=w441:refnum<vi>, error out=w442:errorcluster)  [unwired: 2 in, 3 out]
      n229 = case shown="No Error" w442 {
        tunnel: w441 -> [w452 _]
        frame No Error {
          n230 = call "CRYGet Boolean Reference.vi"("Label Name"="bMsg", "VI Refnum"=w452) -> ("Exist?"=w450:bool, "Boolean Ref"=w449:refnum<vi>)  [unwired: 7 in, 1 out]
          n231 = case shown="True" w450 {
            tunnel: w449 -> [_ w454]
            frame False {
            }
            frame True {
              n232 = property class="Bool"(reference=w454, "Val(Sgnl)"=TRUE) -> ()  [unwired: 1 in, 2 out]
            }
          }
        }
        frame Error {
        }
      }
    }
  }
